vi "Check Distributed Error Manager Status.vi"(8 "error in (no error)":errorcluster, 11 "Local Error Manager in":refnum<class "Local Error Manager.lvclass">) -> (0 "error out":errorcluster, 2 "uService found?":bool, 3 "Local Error Manager out":refnum<class "Local Error Manager.lvclass">)   [LabVIEW 2020, in "TALOS.lvlib" / "Error Manager.lvlib" / "Local Error Manager.lvclass"]
uses:
  Local Error Manager.lvclass
  Local Error Manager.lvclass/Local Error Manager.ctl
  Classes/Distributed uService Map/Distributed uService Map.lvclass
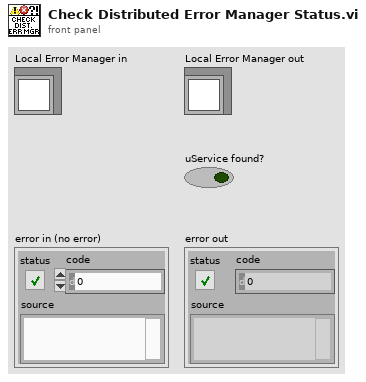
[diagram p1: front panel]
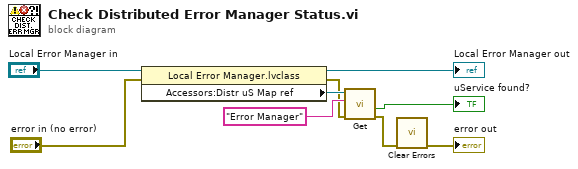
[diagram p0: block diagram]
diagram:
  n1 = property class="Local Error Manager.lvclass"(reference="Local Error Manager in", error in="error in (no error)") -> (reference out=→"Local Error Manager out":refnum<class "Local Error Manager.lvclass">, error out=w2:errorcluster, "Accessors:Distr uS Map ref"=w5:refnum<data-value>)
  n2 = call "Get.vi"("error in (no error)"=w2, "uService ID"="Error Manager", "Distr uS Map ref in"=w5) -> ("error out"=w8:errorcluster, "uService found?"=→"uService found?":bool)  [unwired: 5 in, 2 out]
  n3 = call <vilib>:"Clear Errors.vi"("error in (no error)"=w8) -> ("error out"=→"error out":errorcluster)  [unwired: 5 in, 1 out]
